vi "Write productos.vi"(8 "error in (no error)":errorcluster, 11 "Productos":T1(array[cluster])) -> (0 "error out":errorcluster)   [LabVIEW 2020, in "Config.lvlib"]
uses:
  Config.lvlib
  <vilib>/Utility/sysdir.llb/System Directory Type.ctl
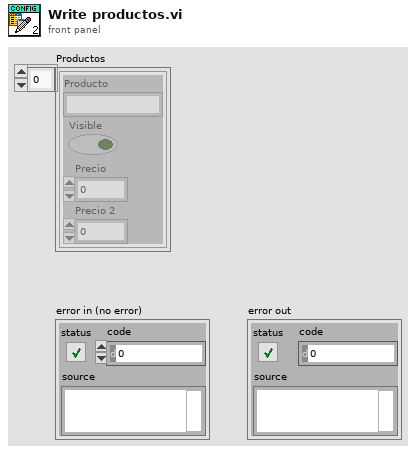
[diagram p1: front panel]
types:
  T1 = cluster{"Producto":string, "Visible":bool, "Precio":dbl, "Precio 2":dbl}[]
  T2 = typedef "System Directory Type.ctl" = i32
  T3 = enum16{"open", "replace", "create", "open or create", "replace or create", "replace or create with confirmation"}
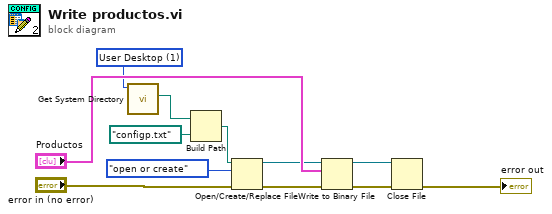
[diagram p0: block diagram]
diagram:
  w10 = T2 1 items=["User Home"=0, "User Desktop"=1, "User Documents"=2, "User Application Data"=3, "User Preferences"=4, "User Temporary"=5, "Public Documents"=6, "Public Application Data"=7, "Public Preferences"=8, "Public Cache"=13, "System Core Libraries"=9, "System Installed Libraries"=10, "Application Files"=11, "Boot Volume Root"=12] ("system directory type")
  n1 = call <vilib>:"Get System Directory.vi"("system directory type"=w10) -> ("system directory"=w3:path)  [unwired: 10 in]
  n2 = Build Path(base path=w3, name or relative path=path "configp.txt") -> (appended path=w5:path)
  n3 = Open/Create/Replace File(file path (use dialog)=w5, error in="error in (no error)", operation (0:open)=T3."open or create") -> (refnum out=w1:refnum<file>, error out=w6:errorcluster)  [unwired: 3 in, 1 out]
  n4 = Write to Binary File(file (use dialog)=w1, data="Productos", error in=w6) -> (refnum out=w8:refnum<file>, error out=w7:errorcluster)  [unwired: 3 in, 1 out]
  n5 = Close File(refnum=w8, error in=w7) -> (error out=→"error out":errorcluster)  [unwired: 1 out]
